vi "6. 读取：文件中的 传感数据 数组.vi"(9 "数据文件名":string="1_第1个设计的data.txt") -> (2 "解析出的 浮点数据":dbl[](array[numeric]) format="%#_13g", 3 "数据点个数":i32)   [LabVIEW 2018]
panel:
  out "路径拆分出 文件名":string="6. 读取：文件中的 传感数据 数组.vi"
  out "正则匹配出 文件名":string="6. 读取：文件中的 传感数据 数组.vi"
  out "数据内容":string="-202.941\t-355.809\t-351.030\t-351.542\t-233.364\t-48.687\t-12.239\t-60.558\t11.939\t62.763\t34.119\t9.283\t-11.175\t-8.096\t6.828\t-37.301\t144.635\t383.052\t321.309\t179.830\t186.766\t569.798\t538.521\t458.801\t373.879\t215.082\t285.410\t464.448\t417.257\t368.603\t374.326\t265.172\t88.523\t-28.345\t-87.013\t67.492\t-95.325\t-330.438\t-379.049\t-439.371\t-629.177\t-607.368\t-488.816\t-513.282\t-535.394\t-600.427\t-604.762\t-619.188\t-630.121\t-478.664\t-205.899\t-152.083\t-354.631\t-604.499\t-648.062\t-479.680\t-202.514\t-78.036\t-8.219\t12.788\t-169.698\t-335.386\t-417.927\t-707.886\t-756.774\t-617.238\t-578.124\t-666.259\t-582.386\t-305.378\t-91.295\t-72.732\t-267.714\t-452.963\t-270.728\t-359.300\t-467.233\t-490.112\t-475.920\t-405.085\t-408.997\t-446.158\t-526.189\t-528.641\t-375.833\t-239.370\t-478.404\t-684.103\t-334.942\t-48.136\t-148.680\t-347.152\t-560.068\t-655.672\t-586.064\t-579.564\t-646.599\t90.378\t333.755\t253.580\t-501.259\t-724.685\t-760.432\t-707.358\t-756.521\t-865.547\t-839.758\t-691.483\t-725.474\t-891.729\t-965.794\t-801.608\t-587.583\t-380.275\t-289.164\t-435.097\t-677.359\t-845.939\t-966.098\t-1005.301\t-988.373\t-1133.712\t-1279.165\t-1399.369\t-1345.837\t-1325.034\t-1575.940\t-1652.237\t-1511.900\t-1329.997\t-1223.109\t-1342.361\t-1462.537\t-1296.857\t-1020.057\t-890.515\t-608.331\t-598.654\t-870.887\t-977.931\t-844.751\t-830.517\t-928.307\t-932.170\t-872.589\t-890.702\t-1003.379\t-1252.310\t-1533.526\t-1715.273\t-1965.379\t-2538.347\t-2574.859\t-2420.588\t-2462.374\t-2605.870\t-2719.697\t-2589.339\t-2495.765\t-2626.198\t-2485.273\t-1857.532\t-519.230\t-220.129\t17.388\t68.063\t70.525\t32.204\t16.718\t31.853\t3.212\t-4.289\t-33.592\t-46.358\t-23.139\t-17.206\t-104.447\t-116.858\t-50.367\t-63.745\t-89.521\t-82.958\t-68.962\t-52.998\t-68.305\t-76.710\t-21.388\t-21.374\t-37.039\t-12.543\t23.919\t117.226\t-245.193\t-43.703\t-17.426\t-34.176\t14.326\t81.720\t114.510\t103.697\t87.883\t35.822\t22.662\t30.951\t54.744\t25.821\t220.429\t132.470\t25.815\t-41.620\t-41.208\t-8.026\t-10.581\t-37.867\t-35.647\t-4.923\t4.767\t-52.570\t-103.478\t-101.351\t-68.378\t-73.109\t-89.961\t-68.574\t-27.236\t12.509\t58.901\t136.774\t188.499\t223.172\t215.127\t147.128\t114.945\t-16.034\t-92.421\t-51.277\t-19.261\t-10.160\t-2.484\t-33.824\t-79.029\t-75.589\t-29.359\t-33.568\t-59.604\t-89.400\t-134.999\t-107.503\t-51.062\t-16.680\t20.737\t-3.836\t-40.283\t-21.838\t11.963\t-22.829\t-52.723\t-1.232\t33.509\t40.713\t-37.539\t-30.330\t41.759\t78.330\t46.006\t46.360\t33.506\t2.776\t-42.750\t-28.540\t-32.576\t-45.067\t-27.031\t-113.889\t-32.266\t-58.842\t-58.549\t-52.033\t-44.922"
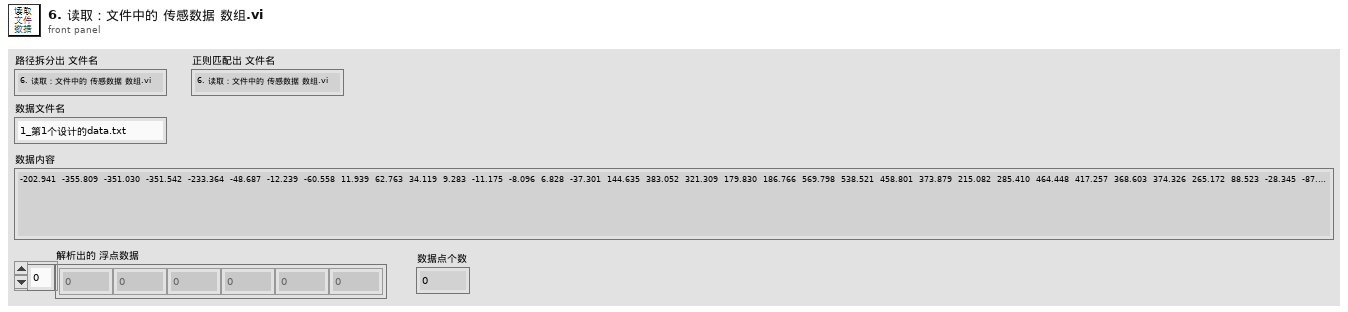
[diagram p1: front panel]
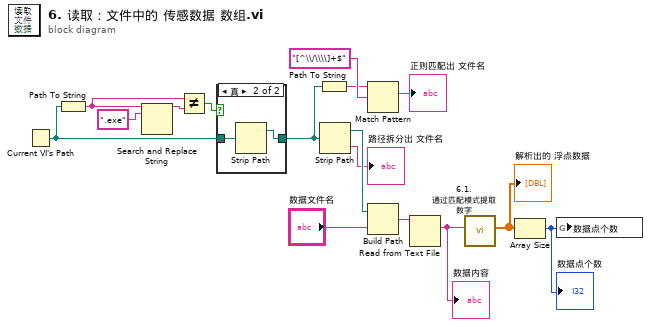
[diagram p0: block diagram]
diagram:
  n1 = Current VI's Path() -> (path=w4:path)
  n2 = Path To String(path=w4) -> (string=w6:string)
  n3 = Search and Replace String(input string=w6, search string=".exe") -> (result string=w7:string)  [unwired: 6 in, 3 out]
  n4 = Not Equal?(x=w6, y=w7) -> (x != y?=w5:bool)
  n5 = case shown="真" w5 {
    tunnel: w4 -> [w17 w19]
    tunnel: [w17 w18] -> w1
    frame False {
    }
    frame True {
      n6 = Strip Path(path=w19) -> (stripped path=w18:path)  [unwired: 1 out]
    }
  }
  n7 = Path To String(path=w1) -> (string=w13:string)
  n8 = Strip Path(path=w1) -> (stripped path=w3:path, name=→"路径拆分出 文件名":string)
  n9 = Match Pattern(string=w13, regular expression="[^\\/\\\\]+$") -> (match substring=→"正则匹配出 文件名":string)  [unwired: 1 in, 3 out]
  n10 = Build Path(base path=w3, name or relative path="数据文件名") -> (appended path=w12:path)
  n11 = Read from Text File(file (use dialog)=w12) -> (text=w16:string)  [unwired: 3 in, 3 out]
  "数据内容" <- w16
  n12 = call "6.1. 通过匹配模式提取数字.vi"("字符串"=w16) -> ("提取的数字"=w10:dbl[])  [unwired: 10 in]
  "解析出的 浮点数据" <- w10
  n13 = Array Size(array=w10) -> (size(s)=w9:i32)
  "数据点个数" <- w9
  n14 = global write "全局变量：数据点个数.vi" "数据点个数"(w9) -> ()
